vi "仪器启动命令.vi"(8 "error in (no error)":errorcluster caption="错误输入（无错误）", 10 "测试模式":enum16{"水样测试", "加标回收"}(ring), 11 "参数":enum16{"氨氮", "总磷", "总氮", "CODMn", "CODcr"}(ring)) -> (0 "error out":errorcluster caption="错误输出")   [LabVIEW 2016, in "质控单元.lvlib"]
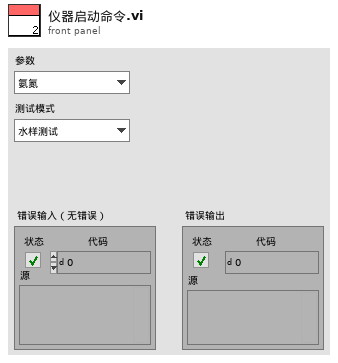
[diagram p1: front panel]
types:
  T1 = cluster{"站号":u16, "量程切换":enum32{"H", "L", "AUTO"}, "控制命令":enum16{"启动测量", "标样核查", "零点核查", "跨度核查", "空白测试", "平行样测试", "加标回收", "空白校准", "标样校准", "初始化（清洗）", "停止测试", "仪器重启", "校时", "模式设置", "测量间隔设置"}, "模式设置":enum16{"待机", "连续模式", "周期模式", "定点模式", "受控模式", "手动模式"}, "测量间隔":u16}
  T2 = enum16{"启动测量", "标样核查", "零点核查", "跨度核查", "空白测试", "平行样测试", "加标回收", "空白校准", "标样校准", "初始化（清洗）", "停止测试", "仪器重启", "校时", "模式设置", "测量间隔设置"}
  T3 = cluster{"测量模式":enum16{"水样测量", "标样核查", "零点核查", "跨度核查", "空白测试", "加标回收", "平行样", "校零", "校标"}}
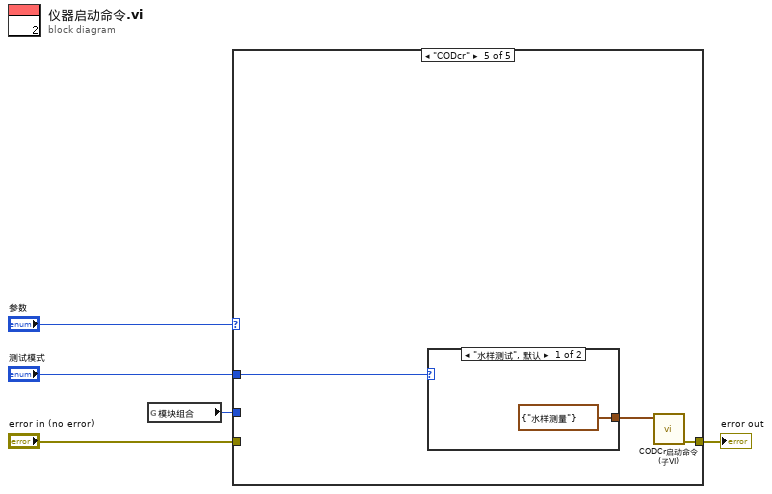
[diagram p0: block diagram]
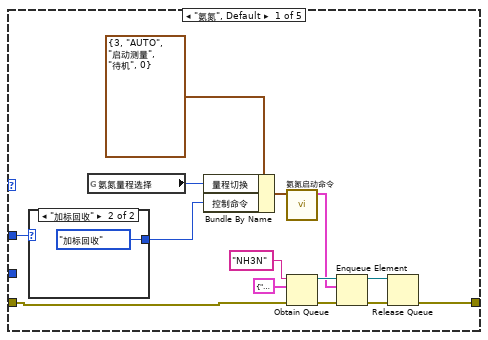
[diagram p2: hidden frame]
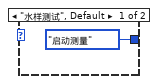
[diagram p3: hidden frame]
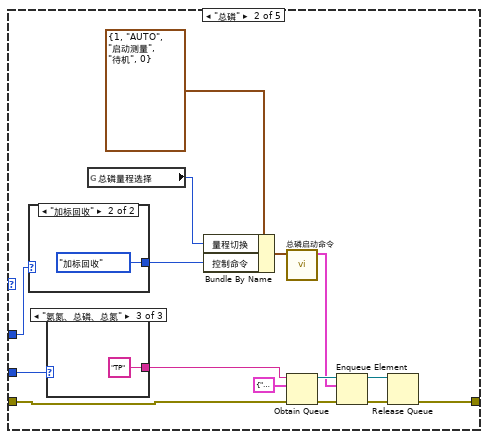
[diagram p4: hidden frame]
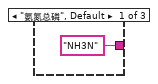
[diagram p5: hidden frame]
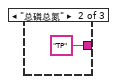
[diagram p6: hidden frame]
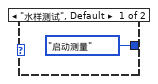
[diagram p7: hidden frame]
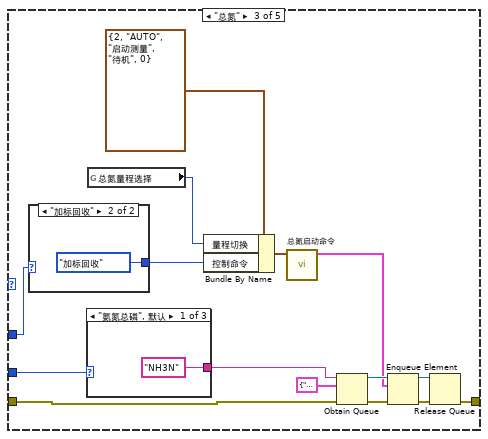
[diagram p8: hidden frame]
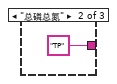
[diagram p9: hidden frame]
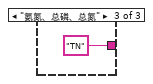
[diagram p10: hidden frame]
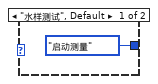
[diagram p11: hidden frame]
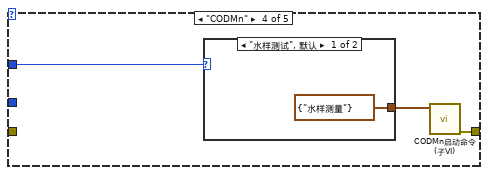
[diagram p12: hidden frame]
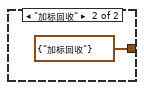
[diagram p13: hidden frame]
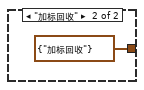
[diagram p14: hidden frame]
diagram:
  n1 = global read "断电保存全局.vi" "模块组合"() -> (w1:enum16{"氨氮总磷", "总磷总氮", "氨氮、总磷、总氮"})
  n2 = case shown="\"CODcr\"" "参数" {
    tunnel: "测试模式" -> [w8 w25 w44 w62 w68]
    tunnel: "error in (no error)" -> [w7 w26 w47 _ _]
    tunnel: [w6 w27 w48 w63 w67] -> w2
    tunnel: w1 -> [_ w23 w43 _ _]
    frame "氨氮", Default {
      n3 = case shown="\"加标回收\"" w8 {
        tunnel: [T2."启动测量" ("控制命令") T2."加标回收" ("控制命令")] -> w17
        frame "水样测试", Default {
        }
        frame "加标回收" {
        }
      }
      n4 = global read "断电保存全局.vi" "氨氮量程选择"() -> (w16:enum32{"H", "L", "AUTO"})
      n5 = Bundle By Name(cluster=T1 {"站号"=3, "量程切换"=enum."AUTO", "控制命令"=enum."启动测量", "模式设置"=enum."待机", "测量间隔"=0} ("参数"), "量程切换"=w16, "控制命令"=w17) -> (w13:T1)
      n6 = call "氨氮启动命令.vi"("参数"=w13) -> ("启动命令"=w11:cluster{"命令":string, "data":variant})  [unwired: 10 in]
      n7 = Obtain Queue(name (unnamed)="NH3N" ("名称（未命名）"), element data type=cluster{"命令":string, "data":variant} {"命令"="", "data"=variant}, error in (no error)=w7) -> (queue out=w14:refnum<queue>, error out=w15:errorcluster)  [unwired: 2 in, 1 out]
      n8 = Enqueue Element(queue=w14, element=w11, error in (no error)=w15) -> (queue out=w18:refnum<queue>, error out=w19:errorcluster)  [unwired: 1 in, 1 out]
      n9 = Release Queue(queue=w18, error in (no error)=w19) -> (error out=w6:errorcluster)  [unwired: 1 in, 2 out]
    }
    frame "总磷" {
      n10 = case shown="\"加标回收\"" w25 {
        tunnel: [T2."启动测量" ("控制命令") T2."加标回收" ("控制命令")] -> w24
        frame "水样测试", Default {
        }
        frame "加标回收" {
        }
      }
      n11 = case shown="\"氨氮、总磷、总氮\"" w23 {
        tunnel: ["NH3N" ("名称（未命名）") "TP" ("名称（未命名）") "TP" ("名称（未命名）")] -> w22
        frame "氨氮总磷", Default {
        }
        frame "总磷总氮" {
        }
        frame "氨氮、总磷、总氮" {
        }
      }
      n12 = global read "断电保存全局.vi" "总磷量程选择"() -> (w33:enum32{"H", "L", "AUTO"})
      n13 = Bundle By Name(cluster=T1 {"站号"=1, "量程切换"=enum."AUTO", "控制命令"=enum."启动测量", "模式设置"=enum."待机", "测量间隔"=0} ("参数"), "量程切换"=w33, "控制命令"=w24) -> (w30:T1)
      n14 = call "总磷启动命令.vi"("参数"=w30) -> ("启动命令"=w28:cluster{"命令":string, "data":variant})  [unwired: 10 in]
      n15 = Obtain Queue(name (unnamed)=w22, element data type=cluster{"命令":string, "data":variant} {"命令"="", "data"=variant}, error in (no error)=w26) -> (queue out=w32:refnum<queue>, error out=w36:errorcluster)  [unwired: 2 in, 1 out]
      n16 = Enqueue Element(queue=w32, element=w28, error in (no error)=w36) -> (queue out=w34:refnum<queue>, error out=w35:errorcluster)  [unwired: 1 in, 1 out]
      n17 = Release Queue(queue=w34, error in (no error)=w35) -> (error out=w27:errorcluster)  [unwired: 1 in, 2 out]
    }
    frame "总氮" {
      n18 = case shown="\"加标回收\"" w44 {
        tunnel: [T2."启动测量" ("控制命令") T2."加标回收" ("控制命令")] -> w56
        frame "水样测试", Default {
        }
        frame "加标回收" {
        }
      }
      n19 = case shown="\"氨氮总磷\", 默认" w43 {
        tunnel: ["NH3N" ("名称（未命名）") "TP" ("名称（未命名）") "TN" ("名称（未命名）")] -> w42
        frame "氨氮总磷", Default {
        }
        frame "总磷总氮" {
        }
        frame "氨氮、总磷、总氮" {
        }
      }
      n20 = global read "断电保存全局.vi" "总氮量程选择"() -> (w52:enum32{"H", "L", "AUTO"})
      n21 = Bundle By Name(cluster=T1 {"站号"=2, "量程切换"=enum."AUTO", "控制命令"=enum."启动测量", "模式设置"=enum."待机", "测量间隔"=0} ("参数"), "量程切换"=w52, "控制命令"=w56) -> (w46:T1)
      n22 = call "总氮启动命令.vi"("参数"=w46) -> ("启动命令"=w45:cluster{"命令":string, "data":variant})  [unwired: 10 in]
      n23 = Obtain Queue(name (unnamed)=w42, element data type=cluster{"命令":string, "data":variant} {"命令"="", "data"=variant}, error in (no error)=w47) -> (queue out=w51:refnum<queue>, error out=w55:errorcluster)  [unwired: 2 in, 1 out]
      n24 = Enqueue Element(queue=w51, element=w45, error in (no error)=w55) -> (queue out=w53:refnum<queue>, error out=w54:errorcluster)  [unwired: 1 in, 1 out]
      n25 = Release Queue(queue=w53, error in (no error)=w54) -> (error out=w48:errorcluster)  [unwired: 1 in, 2 out]
    }
    frame "CODMn" {
      n26 = case shown="\"水样测试\", 默认" w62 {
        tunnel: [T3 {"测量模式"=enum."水样测量"} ("启动测量模式") T3 {"测量模式"=enum."加标回收"} ("启动测量模式")] -> w64
        frame "水样测试", Default {
        }
        frame "加标回收" {
        }
      }
      n27 = call "CODMn启动命令 (子VI).vi"("启动测量模式"=w64) -> ("错误输出"=w63:errorcluster)  [unwired: 10 in]
    }
    frame "CODcr" {
      n28 = case shown="\"水样测试\", 默认" w68 {
        tunnel: [T3 {"测量模式"=enum."水样测量"} ("启动测量模式") T3 {"测量模式"=enum."加标回收"} ("启动测量模式")] -> w69
        frame "水样测试", Default {
        }
        frame "加标回收" {
        }
      }
      n29 = call "CODCr启动命令 (子VI).vi"("启动测量模式"=w69) -> ("错误输出"=w67:errorcluster)  [unwired: 10 in]
    }
  }
  "error out" <- w2
